vi "VC840_Close.vi"(8 "error in (no error)":errorcluster, 11 "VISA resource name":refnum<visa-resource-name>) -> (0 "error out":errorcluster)   [LabVIEW 2010]
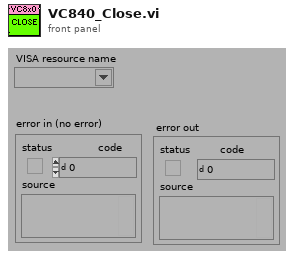
[diagram p1: front panel]
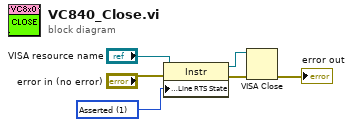
[diagram p0: block diagram]
diagram:
  w6 = i16 1 items=["Unknown"=-1, "Unasserted"=0, "Asserted"=1] ("Modem Line Settings:Line RTS State")
  n1 = property class="Instr"(reference="VISA resource name", error in="error in (no error)", "Serial Settings:Modem Line Settings:Line RTS State"=w6) -> (reference out=w4:refnum<visa-resource-name>, error out=w5:errorcluster)
  n2 = VISA Close(VISA resource name=w4, error in (no error)=w5) -> (error out=→"error out":errorcluster)
